vi "Test Write Function Blocks.vi"(11 "TwinCAT ADS in":refnum<class "TwinCAT ADS.lvclass">) -> (3 "TwinCAT ADS out":refnum<class "TwinCAT ADS.lvclass">)   [LabVIEW 2018]
uses:
  TwinCAT ADS Class/TwinCAT ADS.lvclass
  Controls/FB_Simple.ctl
  Controls/FB_Packed.ctl
  Controls/FB_Complex.ctl
  Controls/ST_Complex.ctl
  Controls/Enum.ctl
  Controls/ST_Simple.ctl
  Controls/ST_Packed.ctl
  9c00ac5c-6d02-4872-9b05-56c396959dcd.vi
  23fdef96-acda-4c8c-ba2d-722c4e2ed0c7.vi
  67abcce4-d906-4956-a77e-4a47c9dde040.vi
  4259b641-f1d6-43a8-a936-771a1071bc54.vi
  1c9d6336-4ba4-42a9-89aa-e685de34db9f.vi
  903064a7-6281-4536-8159-57f8726da337.vi
  TwinCAT ADS Class/VIs/Data/Read.vi
  <vilib>/addons/_JKI Toolkits/Caraya/classes/Assert/Assert True.vi
  <vilib>/addons/_JKI Toolkits/Caraya/classes/Test/Test.lvclass
  <vilib>/addons/_JKI Toolkits/Caraya/classes/Assert/Assert.lvclass
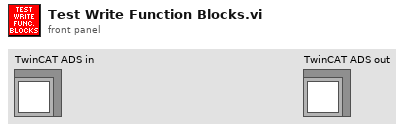
[diagram p1: front panel]
types:
  T1 = typedef "FB_Complex.ctl" = cluster{"_fMember":dbl, "_stMember":T2, "_fbSimpleMember":T6, "_fbPackedMember":T7}
  T2 = typedef "ST_Complex.ctl" = cluster{"bMember":bool, "eMember":T3, "stSimpleMember":T4, "stPackedMember":T5, "FB_Simple":T6, "arrfMember":dbl[]}
  T3 = typedef "Enum.ctl" = enum16{"Member 0", "Member 1", "Member 2"}
  T4 = typedef "ST_Simple.ctl" = cluster{"bMember":bool, "dtMember":timestamp, "nMember":i32}
  T5 = typedef "ST_Packed.ctl" = cluster{"bMember":bool, "dtMember":timestamp, "fMember":dbl}
  T6 = typedef "FB_Simple.ctl" = cluster{"_bMember":bool, "_nMember":i32, "_sMember":string}
  T7 = typedef "FB_Packed.ctl" = cluster{"bMember":bool, "nMember":i32, "sMember":string}
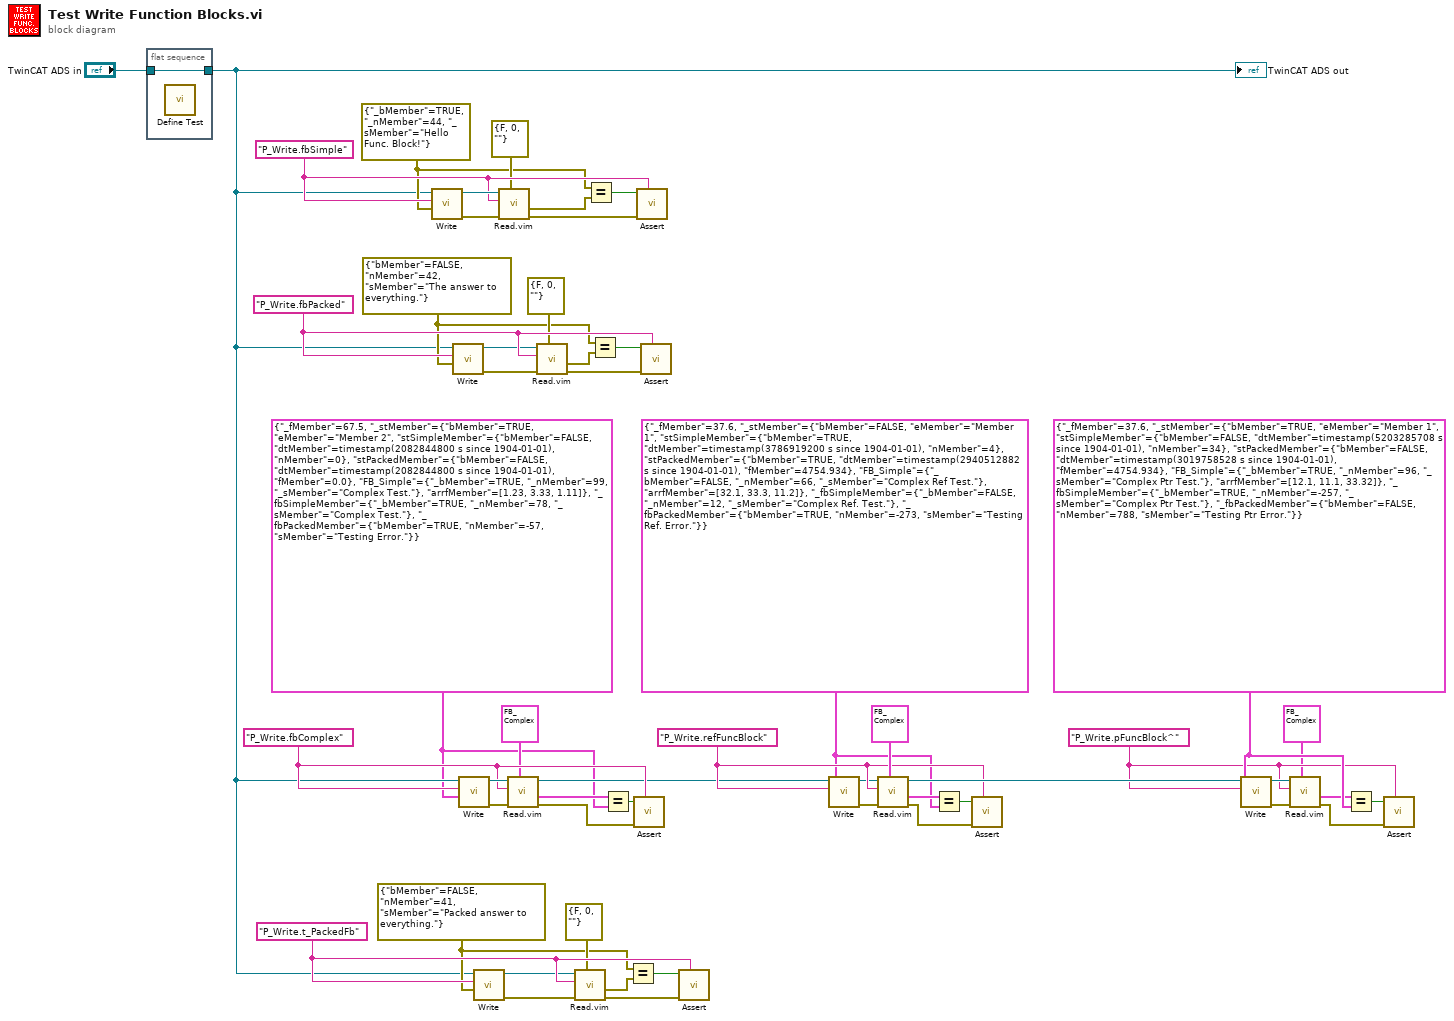
[diagram p0: block diagram]
diagram:
  w8 = T1 {"_fMember"=37.6, "_stMember"={"bMember"=TRUE, "eMember"=enum."Member 1", "stSimpleMember"={"bMember"=FALSE, "dtMember"=timestamp(5203285708 s since 1904-01-01), "nMember"=34}, "stPackedMember"={"bMember"=FALSE, "dtMember"=timestamp(3019758528 s since 1904-01-01), "fMember"=4754.934}, "FB_Simple"={"_bMember"=TRUE, "_nMember"=96, "_sMember"="Complex Ptr Test."}, "arrfMember"=[12.1, 11.1, 33.32]}, "_fbSimpleMember"={"_bMember"=TRUE, "_nMember"=-257, "_sMember"="Complex Ptr Test."}, "_fbPackedMember"={"bMember"=FALSE, "nMember"=788, "sMember"="Testing Ptr Error."}} ("Value")
  w2 = "P_Write.pFuncBlock^" ("Symbol Name")
  w9 = T1 {"_fMember"=37.6, "_stMember"={"bMember"=FALSE, "eMember"=enum."Member 1", "stSimpleMember"={"bMember"=TRUE, "dtMember"=timestamp(3786919200 s since 1904-01-01), "nMember"=4}, "stPackedMember"={"bMember"=TRUE, "dtMember"=timestamp(2940512882 s since 1904-01-01), "fMember"=4754.934}, "FB_Simple"={"_bMember"=FALSE, "_nMember"=66, "_sMember"="Complex Ref Test."}, "arrfMember"=[32.1, 33.3, 11.2]}, "_fbSimpleMember"={"_bMember"=FALSE, "_nMember"=12, "_sMember"="Complex Ref. Test."}, "_fbPackedMember"={"bMember"=TRUE, "nMember"=-273, "sMember"="Testing Ref. Error."}} ("Value")
  w18 = "P_Write.refFuncBlock" ("Symbol Name")
  w21 = T7 {"bMember"=FALSE, "nMember"=41, "sMember"="Packed answer to everything."} ("FB_Packed")
  w28 = "P_Write.t_PackedFb" ("Symbol Name")
  w11 = T1 {"_fMember"=67.5, "_stMember"={"bMember"=TRUE, "eMember"=enum."Member 2", "stSimpleMember"={"bMember"=FALSE, "dtMember"=timestamp(2082844800 s since 1904-01-01), "nMember"=0}, "stPackedMember"={"bMember"=FALSE, "dtMember"=timestamp(2082844800 s since 1904-01-01), "fMember"=0.0}, "FB_Simple"={"_bMember"=TRUE, "_nMember"=99, "_sMember"="Complex Test."}, "arrfMember"=[1.23, 3.33, 1.11]}, "_fbSimpleMember"={"_bMember"=TRUE, "_nMember"=78, "_sMember"="Complex Test."}, "_fbPackedMember"={"bMember"=TRUE, "nMember"=-57, "sMember"="Testing Error."}} ("Value")
  w30 = T7 {"bMember"=FALSE, "nMember"=42, "sMember"="The answer to everything."} ("FB_Packed")
  w32 = T6 {"_bMember"=TRUE, "_nMember"=44, "_sMember"="Hello Func. Block!"} ("FB_Simple")
  w42 = "P_Write.fbPacked" ("Symbol Name")
  w34 = "P_Write.fbComplex" ("Symbol Name")
  w43 = "P_Write.fbSimple" ("Symbol Name")
  n1 = flat-sequence {
    tunnel: "TwinCAT ADS in" -> [w53]
    tunnel: [w53] -> w20
    frame #0 {
      n2 = call <vilib>:"Define Test.vi"() -> ()  [unwired: 10 in, 2 out]
    }
  }
  n3 = call "Write.vi"("Value"=w32, "Symbol Name"=w43, "TwinCAT ADS in"=w20) -> ("error out"=w49:errorcluster, "TwinCAT ADS out"=w50:refnum<class "TwinCAT ADS.lvclass">)  [unwired: 7 in]
  n4 = call "Write.vi"("Value"=w30, "Symbol Name"=w42, "TwinCAT ADS in"=w20) -> ("error out"=w38:errorcluster, "TwinCAT ADS out"=w37:refnum<class "TwinCAT ADS.lvclass">)  [unwired: 7 in]
  n5 = call "Write.vi"("Value"=w11, "Symbol Name"=w34, "TwinCAT ADS in"=w20) -> ("error out"=w48:errorcluster, "TwinCAT ADS out"=w47:refnum<class "TwinCAT ADS.lvclass">)  [unwired: 7 in]
  n6 = call "Write.vi"("Value"=w21, "Symbol Name"=w28, "TwinCAT ADS in"=w20) -> ("error out"=w24:errorcluster, "TwinCAT ADS out"=w23:refnum<class "TwinCAT ADS.lvclass">)  [unwired: 7 in]
  n7 = call "Read.vim"("Type"=T6 {"_bMember"=FALSE, "_nMember"=0, "_sMember"=""} ("FB_Simple"), "error in (no error)"=w49, "Symbol Name"=w43, "TwinCAT ADS in"=w50) -> ("error out"=w46:errorcluster, "Value"=w45:T6)  [unwired: 5 in, 1 out]
  n8 = call "Read.vim"("Type"=T1 {"_fMember"=0.0, "_stMember"={"bMember"=FALSE, "eMember"=enum."Member 0", "stSimpleMember"={"bMember"=FALSE, "dtMember"=timestamp(0 s since 1904-01-01), "nMember"=0}, "stPackedMember"={"bMember"=FALSE, "dtMember"=timestamp(0 s since 1904-01-01), "fMember"=0.0}, "FB_Simple"={"_bMember"=FALSE, "_nMember"=0, "_sMember"=""}, "arrfMember"=[]}, "_fbSimpleMember"={"_bMember"=FALSE, "_nMember"=0, "_sMember"=""}, "_fbPackedMember"={"bMember"=FALSE, "nMember"=0, "sMember"=""}} ("FB_Complex"), "error in (no error)"=w48, "Symbol Name"=w34, "TwinCAT ADS in"=w47) -> ("error out"=w36:errorcluster, "Value"=w12:T1, "TwinCAT ADS out"=w13:refnum<class "TwinCAT ADS.lvclass">)  [unwired: 5 in]
  n9 = call "Read.vim"("Type"=T7 {"bMember"=FALSE, "nMember"=0, "sMember"=""} ("FB_Packed"), "error in (no error)"=w38, "Symbol Name"=w42, "TwinCAT ADS in"=w37) -> ("error out"=w39:errorcluster, "Value"=w40:T7)  [unwired: 5 in, 1 out]
  n10 = call "Read.vim"("Type"=T7 {"bMember"=FALSE, "nMember"=0, "sMember"=""} ("FB_Packed"), "error in (no error)"=w24, "Symbol Name"=w28, "TwinCAT ADS in"=w23) -> ("error out"=w25:errorcluster, "Value"=w26:T7)  [unwired: 5 in, 1 out]
  n11 = Equal?(x=w32, y=w45) -> (x = y?=w44:bool)
  n12 = Equal?(x=w30, y=w40) -> (x = y?=w41:bool)
  n13 = Equal?(x=w12, y=w11) -> (x = y?=w35:bool)
  n14 = Equal?(x=w21, y=w26) -> (x = y?=w27:bool)
  n15 = call-poly <vilib>:"Assert.vi"("Label"=w34, "error in (no error)"=w36, "True?"=w35) -> ()  [unwired: 7 in, 2 out]
  n16 = call-poly <vilib>:"Assert.vi"("Label"=w43, "error in (no error)"=w46, "True?"=w44) -> ()  [unwired: 7 in, 2 out]
  n17 = call-poly <vilib>:"Assert.vi"("Label"=w42, "error in (no error)"=w39, "True?"=w41) -> ()  [unwired: 7 in, 2 out]
  n18 = call-poly <vilib>:"Assert.vi"("Label"=w28, "error in (no error)"=w25, "True?"=w27) -> ()  [unwired: 7 in, 2 out]
  n19 = call "Write.vi"("Value"=w9, "Symbol Name"=w18, "TwinCAT ADS in"=w13) -> ("error out"=w14:errorcluster, "TwinCAT ADS out"=w15:refnum<class "TwinCAT ADS.lvclass">)  [unwired: 7 in]
  n20 = call "Read.vim"("Type"=T1 {"_fMember"=0.0, "_stMember"={"bMember"=FALSE, "eMember"=enum."Member 0", "stSimpleMember"={"bMember"=FALSE, "dtMember"=timestamp(0 s since 1904-01-01), "nMember"=0}, "stPackedMember"={"bMember"=FALSE, "dtMember"=timestamp(0 s since 1904-01-01), "fMember"=0.0}, "FB_Simple"={"_bMember"=FALSE, "_nMember"=0, "_sMember"=""}, "arrfMember"=[]}, "_fbSimpleMember"={"_bMember"=FALSE, "_nMember"=0, "_sMember"=""}, "_fbPackedMember"={"bMember"=FALSE, "nMember"=0, "sMember"=""}} ("FB_Complex"), "error in (no error)"=w14, "Symbol Name"=w18, "TwinCAT ADS in"=w15) -> ("error out"=w16:errorcluster, "Value"=w10:T1, "TwinCAT ADS out"=w52:refnum<class "TwinCAT ADS.lvclass">)  [unwired: 5 in]
  n21 = Equal?(x=w10, y=w9) -> (x = y?=w17:bool)
  n22 = call-poly <vilib>:"Assert.vi"("Label"=w18, "error in (no error)"=w16, "True?"=w17) -> ()  [unwired: 7 in, 2 out]
  n23 = call "Write.vi"("Value"=w8, "Symbol Name"=w2, "TwinCAT ADS in"=w52) -> ("error out"=w6:errorcluster, "TwinCAT ADS out"=w5:refnum<class "TwinCAT ADS.lvclass">)  [unwired: 7 in]
  n24 = call "Read.vim"("Type"=T1 {"_fMember"=0.0, "_stMember"={"bMember"=FALSE, "eMember"=enum."Member 0", "stSimpleMember"={"bMember"=FALSE, "dtMember"=timestamp(0 s since 1904-01-01), "nMember"=0}, "stPackedMember"={"bMember"=FALSE, "dtMember"=timestamp(0 s since 1904-01-01), "fMember"=0.0}, "FB_Simple"={"_bMember"=FALSE, "_nMember"=0, "_sMember"=""}, "arrfMember"=[]}, "_fbSimpleMember"={"_bMember"=FALSE, "_nMember"=0, "_sMember"=""}, "_fbPackedMember"={"bMember"=FALSE, "nMember"=0, "sMember"=""}} ("FB_Complex"), "error in (no error)"=w6, "Symbol Name"=w2, "TwinCAT ADS in"=w5) -> ("error out"=w4:errorcluster, "Value"=w7:T1)  [unwired: 5 in, 1 out]
  n25 = Equal?(x=w7, y=w8) -> (x = y?=w3:bool)
  n26 = call-poly <vilib>:"Assert.vi"("Label"=w2, "error in (no error)"=w4, "True?"=w3) -> ()  [unwired: 7 in, 2 out]
  "TwinCAT ADS out" <- w20
